vi "json_next.vi"(0 "c":string, 5 "text":string, 7 "ch":string, 9 "at":i32, 11 "error in (no error)":errorcluster) -> (6 "text dup":string, 8 "ch out":string, 10 "at out":i32, 15 "error out":errorcluster)   [LabVIEW 2011]
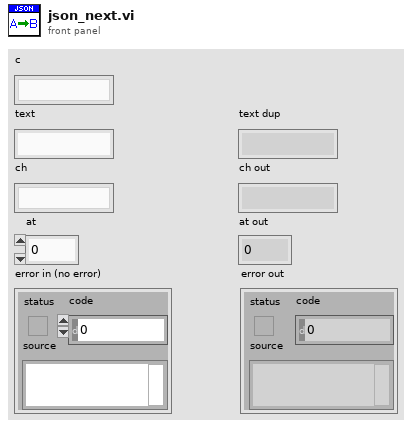
[diagram p1: front panel]
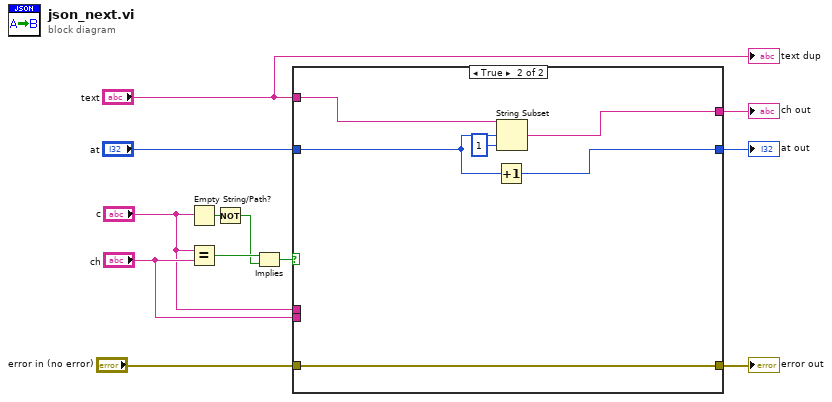
[diagram p0: block diagram]
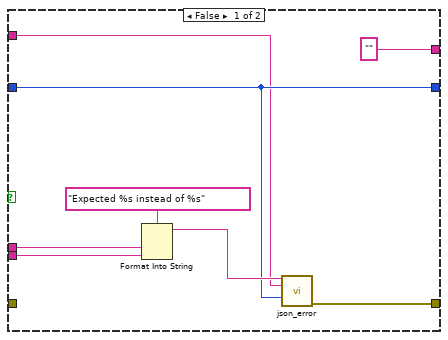
[diagram p2: hidden frame]
diagram:
  n1 = Empty String/Path?(string/path="c") -> (empty?=w12:bool)
  n2 = Equal?(x="c", y="ch") -> (x = y?=w11:bool)
  n3 = Not(x=w12) -> (.not. x?=w10:bool)
  n4 = Implies(1:w10, 2:w11) -> (0:w9:bool)
  n5 = case shown="True" w9 {
    tunnel: "error in (no error)" -> [_ w26]
    tunnel: [w15 w26] -> w7
    tunnel: "at" -> [w14 w24]
    tunnel: "text" -> [w13 w23]
    tunnel: [w14 w21] -> w3
    tunnel: ["" ("text") w22] -> w5
    tunnel: "ch" -> [w18 _]
    tunnel: "c" -> [w17 _]
    frame False {
      n6 = Format Into String(format string="Expected %s instead of %s", w17, w18) -> (resulting string=w16:string)  [unwired: 2 in, 1 out]
      n7 = call "json_error.vi"("m"=w16, "text"=w13, "at"=w14) -> ("error out"=w15:errorcluster)  [unwired: 12 in]
    }
    frame True {
      n8 = Increment(x=w24) -> (x+1=w21:i32)
      n9 = String Subset(string=w23, offset (0)=w24, length (rest)=1 ("length (rest)")) -> (substring=w22:string)
    }
  }
  "at out" <- w3
  "ch out" <- w5
  "error out" <- w7
  "text dup" <- "text"
